vi "proc_cleanup.vi"(8 "error in":errorcluster, 11 "process instance handle in":u32[](array[numeric])) -> (0 "error out":errorcluster, 3 "process instance handle out":u32[](array[numeric]))   [LabVIEW 2012]
doc: "Closes process instance handle. This VI does not terminates the process! It only closes opened handles to it contained in process instance handle structure but it is still required to be called after the process returned exit code otherwise all handles (process, main thread, pies) stays opened."
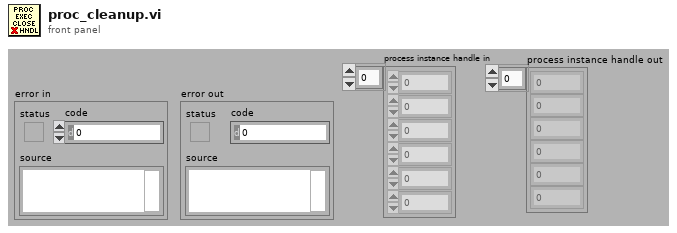
[diagram p1: front panel]
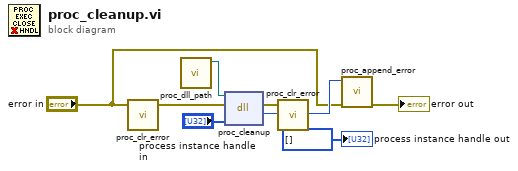
[diagram p0: block diagram]
diagram:
  n1 = call "proc_clr_error.vi"("error in (no error)"="error in") -> ("error out"=w5:errorcluster)  [unwired: 4 in]
  n2 = call "proc_dll_path.vi"() -> ("path out"=w8:path)  [unwired: 10 in, 1 out]
  n3 = dll-call lib="lv_proc.dll" fn="proc_cleanup"(path in=w8, error in=w5, "proc"="process instance handle in") -> (error out=w4:errorcluster, "error"=w6:i32)  [unwired: 2 in, 1 out]
  n4 = call "proc_clr_error.vi"("error in (no error)"=w4) -> ()  [unwired: 4 in, 1 out]
  n5 = call "proc_append_error.vi"("error in"="error in", "code in"=w6) -> ("error out"=→"error out":errorcluster)  [unwired: 8 in, 1 out]
  "process instance handle out" <- u32[] [] ("process instance handle out")
